vi "Do.vi"(8 "error in (no error)":errorcluster, 10 "Actor in":refnum<class "Actor.lvclass">, 11 "update DVR pool from nested actors Msg":refnum<class "update DVR pool from nested actors Msg.lvclass">) -> (0 "error out":errorcluster, 2 "Actor out":refnum<class "Actor.lvclass">)   [LabVIEW 2020, in "Template.lvlib" / "update DVR pool from nested actors Msg.lvclass"]
doc: "This VI delivers the message to the actor by calling the appropriate method(s) on the actor."
uses:
  update DVR pool from nested actors Msg.lvclass
  <vilib>/ActorFramework/Actor/Actor.lvclass
  update DVR pool from nested actors Msg.lvclass/update DVR pool from nested actors Msg.ctl
  template/Template.lvclass
  C:/Program Files/National Instruments/LabVIEW 2020/vi.lib/ActorFramework/Actor/Actor.lvclass
  0c47bd1a-e0b2-4967-91ed-70c0a69e1e3a.vi
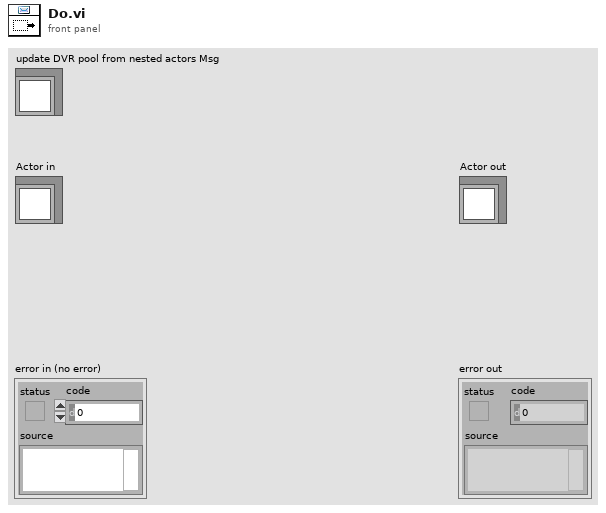
[diagram p1: front panel]
types:
  T1 = typedef "Template.lvlib/Template.lvclass/base actor queues.ctl" = cluster{"DVR Pool":refnum<queue>, "Actor's Data":refnum<queue>}
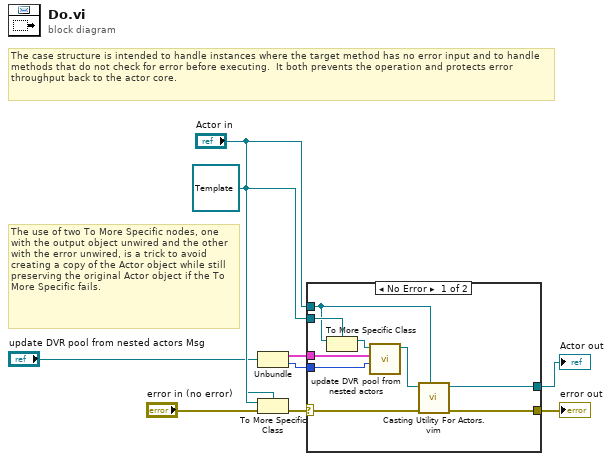
[diagram p0: block diagram]
diagram:
  w4 = refnum<class "Template.lvclass"> refnum ("Actor in")
  # "The use of two To More Specific nodes, one with the output object unwired and the other with the error unwired, is a trick to avoid creating a copy of the Actor object while still preserving the original Actor object if the To More Specific fails."
  # "The case structure is intended to handle instances where the target method has no error input and to handle methods that do not check for error before executing.  It both prevents the operation and protects error throughput back to the actor core."
  n1 = Unbundle("update DVR pool from nested actors Msg") -> (w2:T1, w1:u32)
  n2 = To More Specific Class(target class=w4, reference="Actor in", error in="error in (no error)") -> (error out=w3:errorcluster)  [unwired: 1 out]
  n3 = case shown="No Error" w3 {
    selector: w3 -> [w18 w20]
    tunnel: [w12 w20] -> w9
    tunnel: [w13 w19] -> w8
    tunnel: "Actor in" -> [w15 w19]
    tunnel: w4 -> [w16 _]
    tunnel: w2 -> [w11 _]
    tunnel: w1 -> [w10 _]
    frame No Error {
      n4 = To More Specific Class(target class=w16, reference=w15) -> (specific class reference=w17:refnum<class "Template.lvclass">)  [unwired: 1 in, 1 out]
      n5 = call "update DVR pool from nested actors.vi"("Actor number"=w10, "Base Actor Queues"=w11, "Template in"=w17) -> ("Template out"=w14:refnum<class "Template.lvclass">)  [unwired: 8 in]
      n6 = call "Casting Utility For Actors.vim"("type"=w15, "error in (no error)"=w18, "Actor in"=w14) -> ("error out"=w12:errorcluster, "Actor out"=w13:refnum<class "Actor.lvclass">)  [unwired: 7 in]
    }
    frame Error {
      # "If type check fails, pass the original object out again."
    }
  }
  "error out" <- w9
  "Actor out" <- w8
